vi "动力环境监测系统.vi"() -> ()   [LabVIEW 2016, in "环境动力监测库.lvlib"]
panel:
  in  "权限等级":enum16{"一级权限", "二级权限", "三级权限", "超级权限"}(ring)
  in  "应用环境":enum16{"固定站", "微站", "浮标", "浮船"}(ring)
  in  "单选按钮":enum32{"首页", "设备配置"}(radio)
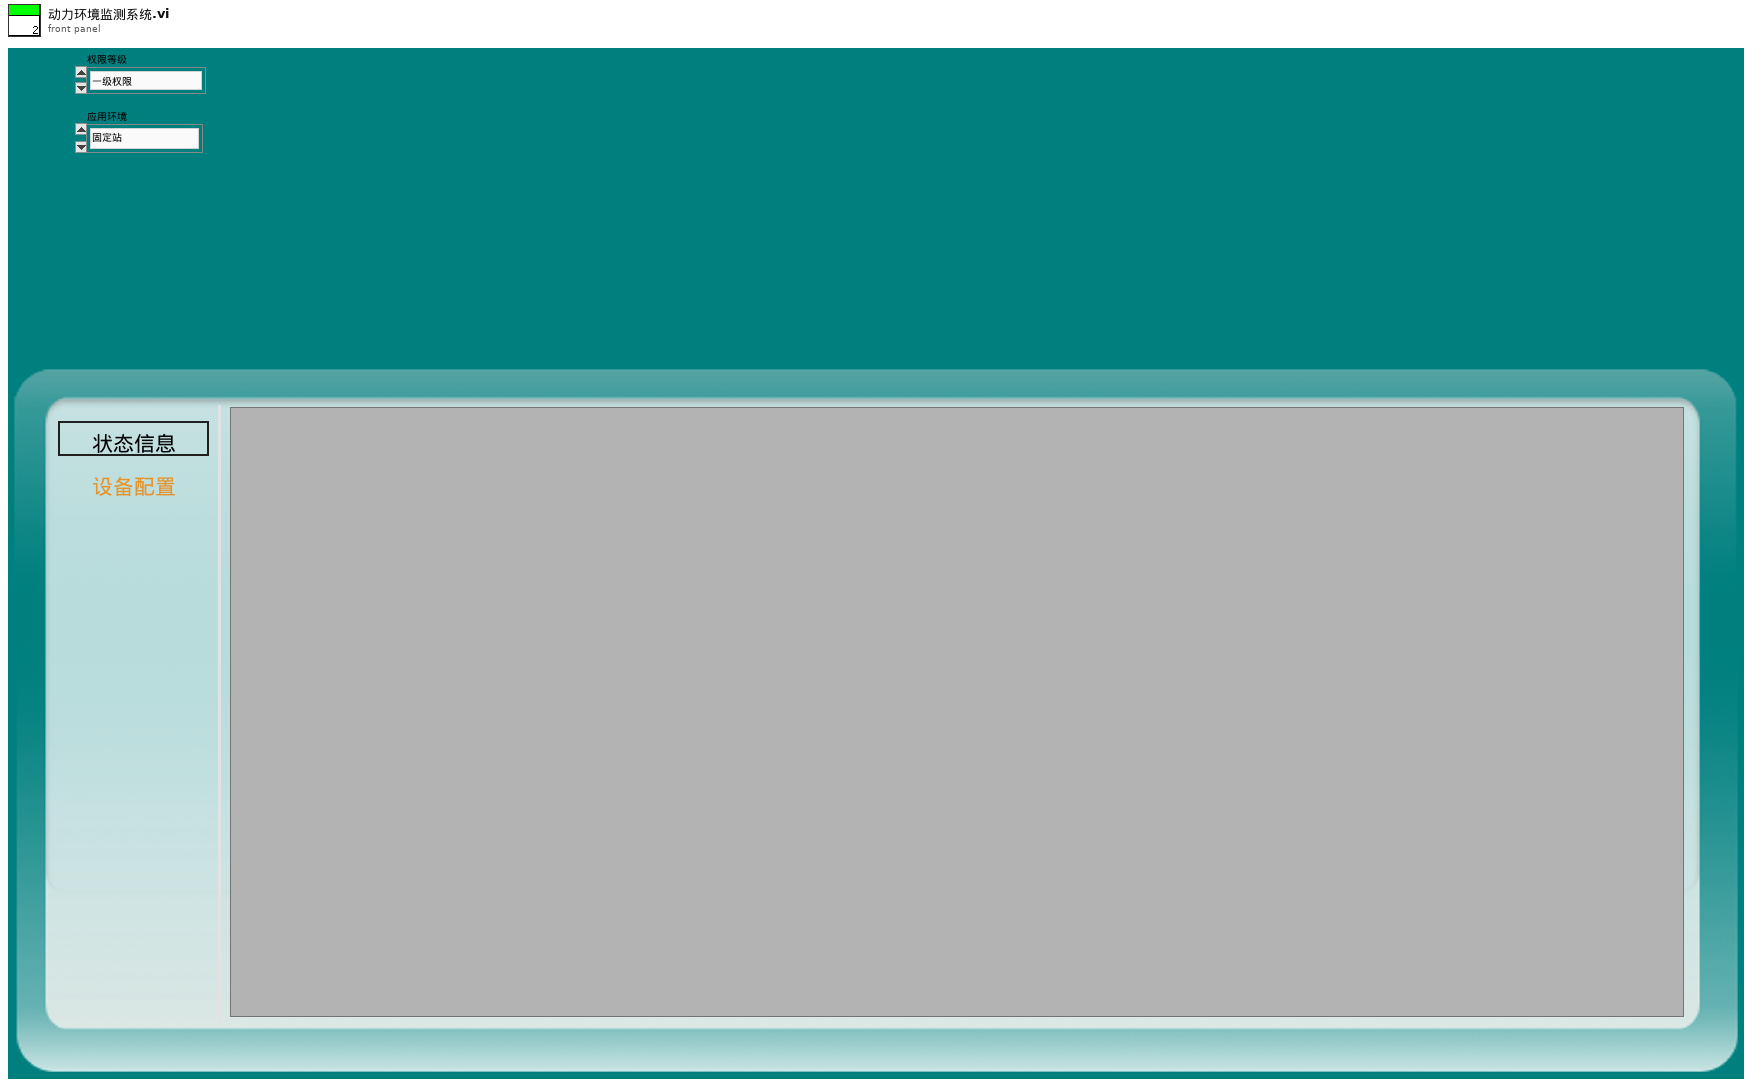
[diagram p1: front panel]
types:
  T1 = enum32{"Bad", "Idle", "Run top level", "Running"}
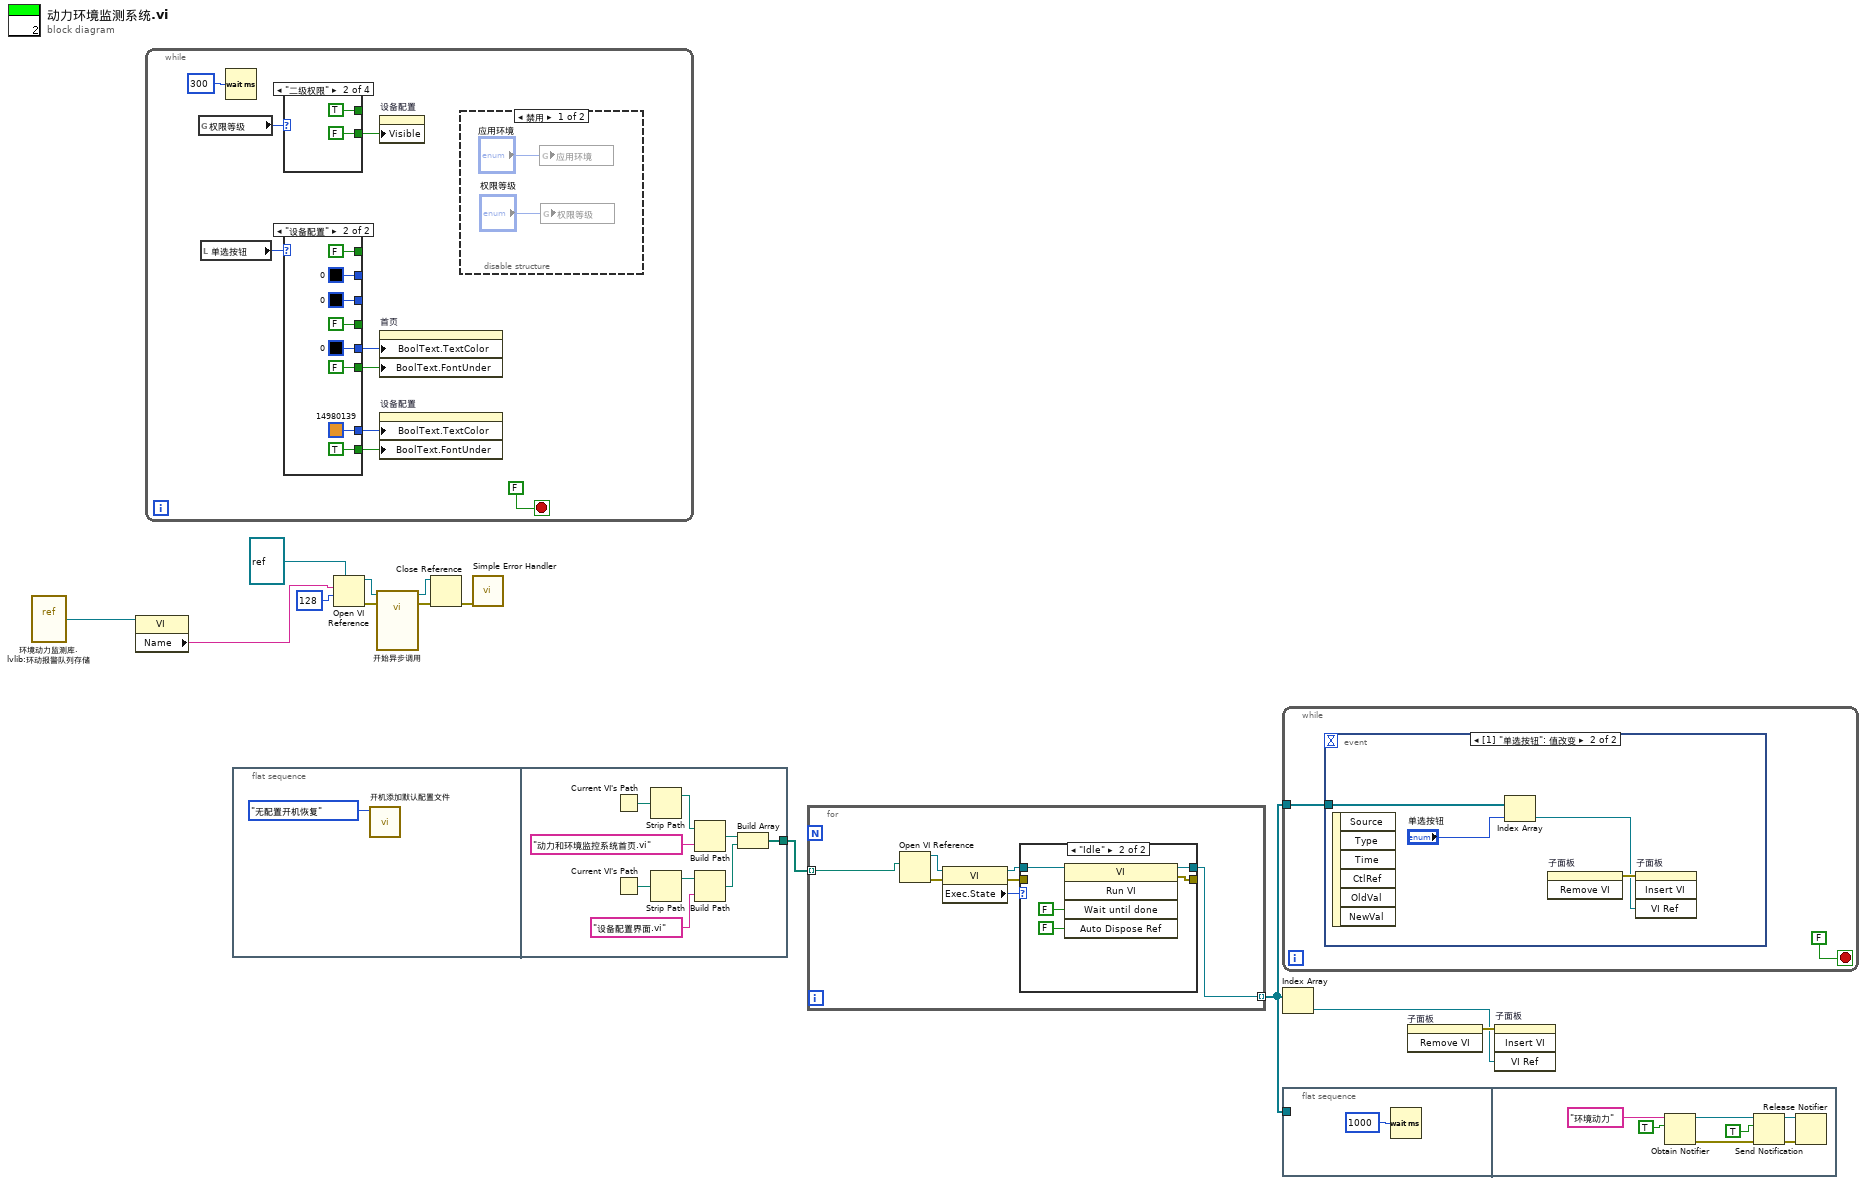
[diagram p0: block diagram]
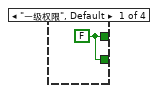
[diagram p3: hidden frame]
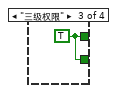
[diagram p4: hidden frame]
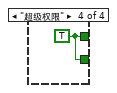
[diagram p5: hidden frame]
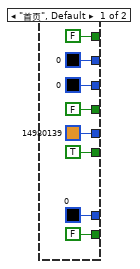
[diagram p6: hidden frame]
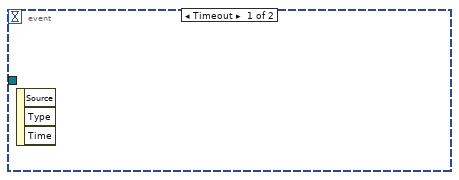
[diagram p7: hidden frame]
diagram:
  n1 = vi-ref "环境动力监测库.lvlib:环动报警队列存储.vi"() -> (w2:refnum<vi>)
  n2 = property class="VI"(reference=w2) -> ("Name"=w1:string)  [unwired: 1 in, 2 out]
  n3 = while {
    stop <- FALSE stop-if-true
    n4 = global read "外部交互全局变量.vi" "权限等级"() -> (w15:enum16{"一级权限", "二级权限", "三级权限", "超级权限"})
    n5 = local read "单选按钮"() -> (w18:enum32{"首页", "设备配置"})
    n6 = Wait (ms)(milliseconds to wait=u32 300 ("等待时间（毫秒）")) -> ()  [unwired: 1 out]
    n7 = case shown="\"二级权限\"" w15 {
      tunnel: [w25 TRUE w28 w29] -> _
      tunnel: [w25 FALSE w28 w29] -> w14
      frame "一级权限", Default {
        w25 = FALSE
      }
      frame "二级权限" {
      }
      frame "三级权限" {
        w28 = TRUE
      }
      frame "超级权限" {
        w29 = TRUE
      }
    }
    n8 = case shown="\"设备配置\"" w18 {
      tunnel: [u32 0 u32 14980139] -> w21
      tunnel: [FALSE ("布尔文本.字体:下划线") TRUE ("布尔文本.字体:下划线")] -> w22
      tunnel: [u32 0 u32 0] -> _
      tunnel: [FALSE ("布尔文本.字体:下划线") FALSE ("布尔文本.字体:下划线")] -> _
      tunnel: [u32 14980139 u32 0] -> w19
      tunnel: [TRUE ("布尔文本.字体:下划线") FALSE ("布尔文本.字体:下划线")] -> w20
      tunnel: [u32 0 u32 0] -> _
      tunnel: [FALSE ("布尔文本.字体:下划线") FALSE ("布尔文本.字体:下划线")] -> _
      frame "首页", Default {
      }
      frame "设备配置" {
      }
    }
    n9 = property on="设备配置" class="Bool (严格)"("Visible"=w14) -> ()  [unwired: 2 in, 2 out]
    n10 = property on="首页" class="Bool (严格)"("BoolText.TextColor"=w19, "BoolText.FontUnder"=w20) -> ()  [unwired: 2 in, 2 out]
    n11 = property on="设备配置" class="Bool (严格)"("BoolText.TextColor"=w21, "BoolText.FontUnder"=w22) -> ()  [unwired: 2 in, 2 out]
    n12 = disable-structure shown="禁用" {
      frame Disabled {
        n13 = global write "外部交互全局变量.vi" "应用环境"("应用环境") -> ()
        n14 = global write "外部交互全局变量.vi" "权限等级"("权限等级") -> ()
      }
      frame Enabled {
      }
    }
  }
  n15 = flat-sequence {
    tunnel: [w55] -> w13
    frame #0 {
      n16 = call "开机添加默认配置文件.vi"("恢复默认方式"=enum16{"无配置开机恢复", "手动恢复"}."无配置开机恢复") -> ()  [unwired: 10 in, 1 out]
    }
    frame #1 {
      n17 = Current VI's Path() -> (path=w54:path)
      n18 = Current VI's Path() -> (path=w48:path)
      n19 = Strip Path(path=w54) -> (stripped path=w53:path)  [unwired: 1 out]
      n20 = Strip Path(path=w48) -> (stripped path=w49:path)  [unwired: 1 out]
      n21 = Build Path(base path=w53, name or relative path="动力和环境监控系统首页.vi" ("名称或相对路径")) -> (appended path=w51:path)
      n22 = Build Path(base path=w49, name or relative path="设备配置界面.vi" ("名称或相对路径")) -> (appended path=w47:path)
      n23 = Build Array(w51, w47) -> (w55:path[])
    }
  }
  n24 = Open VI Reference(type specifier VI Refnum (for type only)=refnum<vi> refnum ("类型说明符VI引用句柄（仅用于类型）"), vi path=w1, options=128 ("选项")) -> (vi reference=w8:refnum<vi>, error out=w10:errorcluster)  [unwired: 3 in]
  n25 = call-by-ref "开始异步调用"(reference=w8, error in=w10) -> (reference out=w7:refnum<vi>, error out=w6:errorcluster)  [unwired: 12 in]
  n26 = Close Reference(reference=w7, error in (no error)=w6) -> (error out=w5:errorcluster)
  n27 = call <vilib>:"Simple Error Handler.vi"("error in (no error)"=w5) -> ()  [unwired: 4 in, 5 out]
  n28 = for {
    tunnel: w13 -> [w57] mode=indexing
    tunnel: [w56] -> w4 mode=indexing
    n29 = Open VI Reference(vi path=w57) -> (vi reference=w60:refnum<vi>, error out=w59:errorcluster)  [unwired: 5 in]
    n30 = property class="VI"(reference=w60, error in=w59) -> (reference out=w61:refnum<vi>, error out=w58:errorcluster, "Exec.State"=w62:T1)
    n31 = case shown="\"Idle\"" w62 {
      tunnel: w61 -> [w64 w67]
      tunnel: [w64 w66] -> w56
      tunnel: [w63 w65] -> _
      tunnel: w58 -> [w63 _]
      frame "Bad", Default {
      }
      frame "Idle" {
        n32 = invoke class="VI" method="Run VI"(reference=w67, "Wait until done"=FALSE ("结束前等待"), "Auto Dispose Ref"=FALSE ("自动销毁引用")) -> (reference out=w66:refnum<vi>, error out=w65:errorcluster)  [unwired: 2 in, 3 out]
      }
    }
  }
  n33 = while {
    tunnel: w4 -> [w70]
    stop <- FALSE stop-if-true
    n34 = event shown="[1] \"单选按钮\": 值改变" {
      selector: _ -> [_ _]
      dyn-events: _ -> [_ _]
      timeout: _ -> [_ _]
      tunnel: w70 -> [_ w74]
      event Timeout {
        n35 = event-data() -> ()  [unwired: 1 in, 3 out]
      }
      event "单选按钮": Value Change {
        n36 = event-data() -> ()  [unwired: 1 in, 6 out]
        n37 = Index Array(array=w74, index="单选按钮") -> (element=w72:refnum<vi>)
        n38 = invoke on="子面板" class="SubPnl" method="Remove VI"() -> (error out=w75:errorcluster)  [unwired: 3 in, 2 out]
        n39 = invoke on="子面板" class="SubPnl" method="Insert VI"(error in=w75, "VI Ref"=w72) -> ()  [unwired: 2 in, 4 out]
      }
    }
  }
  n40 = Index Array(array=w4) -> (element=w3:refnum<vi>)  [unwired: 1 in]
  n41 = flat-sequence {
    tunnel: w4 -> [_]
    frame #0 {
      n42 = Wait (ms)(milliseconds to wait=u32 1000 ("等待时间（毫秒）")) -> ()  [unwired: 1 out]
    }
    frame #1 {
      n43 = Obtain Notifier(name (unnamed)="环境动力" ("名称（未命名）"), notification data type=TRUE) -> (notifier out=w82:refnum<notifier>, error out=w78:errorcluster)  [unwired: 2 in, 1 out]
      n44 = Send Notification(notification=TRUE ("通知"), notifier=w82, error in (no error)=w78) -> (notifier out=w81:refnum<notifier>, error out=w77:errorcluster)
      n45 = Release Notifier(notifier=w81, error in (no error)=w77) -> ()  [unwired: 1 in, 3 out]
    }
  }
  n46 = invoke on="子面板" class="SubPnl" method="Remove VI"() -> (error out=w12:errorcluster)  [unwired: 3 in, 2 out]
  n47 = invoke on="子面板" class="SubPnl" method="Insert VI"(error in=w12, "VI Ref"=w3) -> ()  [unwired: 2 in, 4 out]
